vi "Dhoot_Sealed_side.vi"(0 "Calibrated Image":T3, 1 "Image In":T3(plugin-control), 2 "Centre X":dbl, 3 "Centre Y":dbl, 4 "Ref Edge ROI":T4, 5 "Ref Search Direction":u32(ring)=2 items=["Left to Right", "Right to Left", "Top to Bottom", "Bottom to Top"], 6 "Ref Edge Options":T7={"Edge Polarity"=2, "Kernel Size"=3, "Width"=3, "Minimum Edge Strength"=50.0, "Interpolation Type"=enum."Zero Order", "Data Processing Method"=enum."Average"} {"Edge Polarity" items=["All Edges", "Rising Edges", "Falling Edges"]; "Minimum Edge Strength" format="%.2f"; "Width" step=2; "Kernel Size" step=2}, 7 "error in (no error)":errorcluster, 8 "Meas ROI 1 [Before Transformation]":T2 {"Contours"."Type" items=["No Selection", "Point", "Line", "Rectangle", "Oval", "Polygon", "Freehand Region", "Annulus", "Unused2", "Unused3", "Broken Line", "Freehand Line", "Rotated Rectangle"]}, 9 "Ref Line Options":T5={"Number of Lines"=1, "Type"=enum."Best Edge Rake", "Min. Score"=10.0, "Max. Score"=1000.0, "Orientation"=0.0, "Angle Range"=50.0, "Angle Tolerance"=1.0, "Step Size"=3, "Min. SNR (db)"=0.0, "Min. Points (%)"=25.0, "Hough Iterations"=5} {"Min. Points (%)" min=0.0 max=100.0; "Min. SNR (db)" min=0.0; "Max. Score" min=0.0 max=1024.0; "Min. Score" min=0.0 max=1024.0 step=1.0}, 10 "ROI 1 Step Size":u32=5, 11 "Meas ROI 2 [Before Transformation]":T2 {"Contours"."Type" items=["No Selection", "Point", "Line", "Rectangle", "Oval", "Polygon", "Freehand Region", "Annulus", "Unused2", "Unused3", "Broken Line", "Freehand Line", "Rotated Rectangle"]}, 12 "ROI 1 Scan Direction":u16(ring) items=["Left To Right", "Right To Left", "Top To Bottom", "Bottom To Top"], 13 "ROI 2 Step Size":u32=5, 14 "ROI 1 Process":T9(ring)=enum."Get All Edges", 15 "ROI 2 Scan Direction":u16(ring) items=["Left To Right", "Right To Left", "Top To Bottom", "Bottom To Top"], 16 "ROI 1 Edge Options":T7={"Edge Polarity"=2, "Kernel Size"=3, "Width"=3, "Minimum Edge Strength"=50.0, "Interpolation Type"=enum."Zero Order", "Data Processing Method"=enum."Average"} {"Edge Polarity" items=["All Edges", "Rising Edges", "Falling Edges"]; "Minimum Edge Strength" format="%.2f"; "Width" step=2; "Kernel Size" step=2}, 17 "ROI 2 Process":T9(ring)=enum."Get All Edges", 18 "Overlay Enable":bool, 19 "ROI 2 Edge Options":T7={"Edge Polarity"=2, "Kernel Size"=3, "Width"=3, "Minimum Edge Strength"=50.0, "Interpolation Type"=enum."Zero Order", "Data Processing Method"=enum."Average"} {"Edge Polarity" items=["All Edges", "Rising Edges", "Falling Edges"]; "Minimum Edge Strength" format="%.2f"; "Width" step=2; "Kernel Size" step=2}) -> (21 "Side Length":sgl, 23 "Arrow Overlay lines":T1, 27 "error out":errorcluster)   [LabVIEW 2019, in "Algorithm.lvclass"]
uses:
  FrameworkOverrides/Algorithm.lvclass
  <vilib>/vision/NI_Vision_Development_Module.lvlib
  <vilib>/vision/Measure.llb/Edge Polarity.ctl
  <vilib>/vision/Measure.llb/Edge Options.ctl
  <vilib>/vision/Measure.llb/Straight Edge Process.ctl
  <vilib>/vision/Measure.llb/Straight Edge Options.ctl
  <vilib>/vision/Image Controls.llb/IMAQ Image.ctl
panel:
  out "max value 2":dbl
  out "max value":dbl
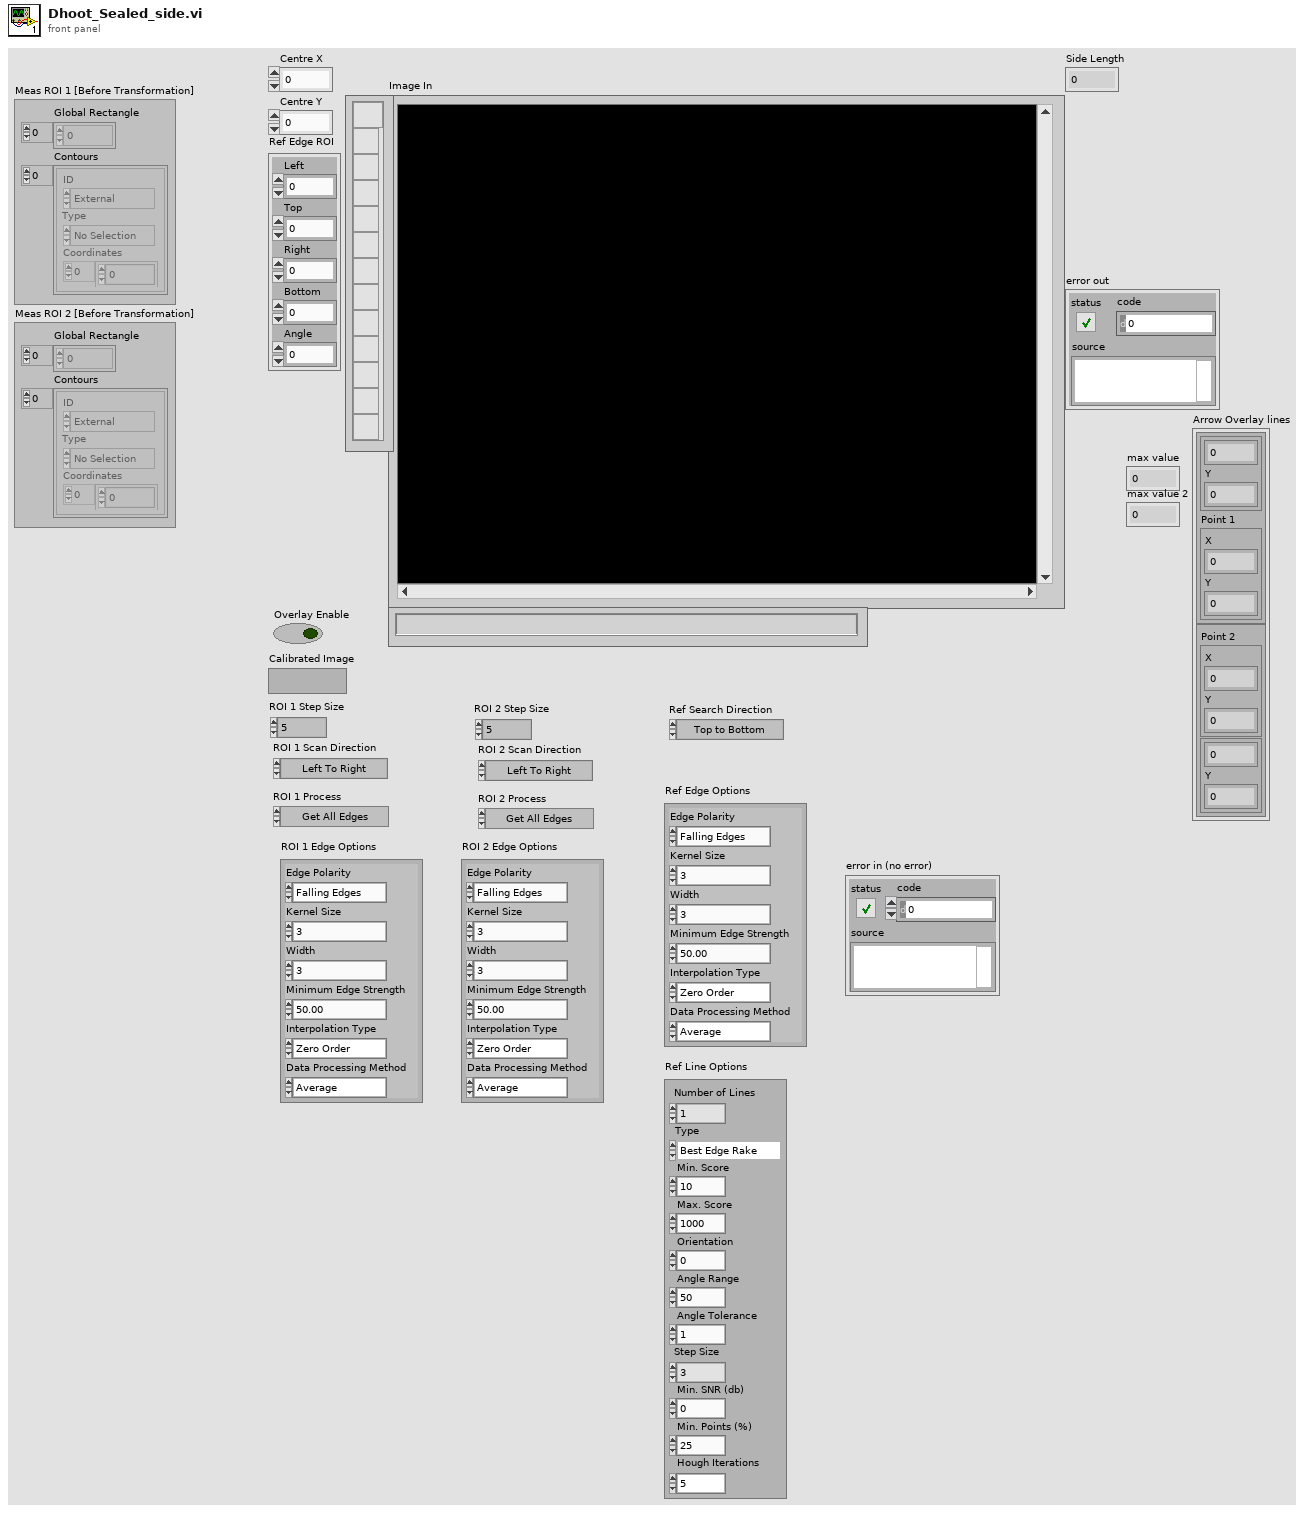
[diagram p1: front panel]
types:
  T1 = cluster{cluster{cluster{sgl, "Y":sgl}, "Point 1":cluster{"X":sgl, "Y":sgl}}, cluster{"Point 2":cluster{"X":sgl, "Y":sgl}, cluster{sgl, "Y":sgl}}}
  T2 = typedef "ROI Descriptor" = cluster{"Global Rectangle":i32[], "Contours":cluster{"ID":enum32{"External", "Internal"}, "Type":u32, "Coordinates":i32[]}[]}
  T3 = typedef "IMAQ Image.ctl" = refnum<image>
  T4 = cluster{"Left":dbl, "Top":dbl, "Right":dbl, "Bottom":dbl, "Angle":dbl}
  T5 = typedef "Straight Edge Options.ctl" = cluster{"Number of Lines":i32, "Type":T6, "Min. Score":dbl, "Max. Score":dbl, "Orientation":dbl, "Angle Range":dbl, "Angle Tolerance":dbl, "Step Size":u32, "Min. SNR (db)":dbl, "Min. Points (%)":dbl, "Hough Iterations":i32}
  T6 = typedef "Straight Edge Process.ctl" = enum32{"First Edge Rake", "Best Edge Rake", "Hough Edge Rake", "First Edge Projection", "Best Edge Projection"}
  T7 = typedef "Edge Options.ctl" = cluster{"Edge Polarity":T8, "Kernel Size":u32, "Width":u32, "Minimum Edge Strength":sgl, "Interpolation Type":enum32{"Zero Order", "Bilinear", "Quadratic", "Cubic", "Bilinear Fixed"}, "Data Processing Method":enum32{"Average", "Median"}}
  T8 = typedef "Edge Polarity.ctl" = u32
  T9 = enum16{"Get First Edge", "Get First + Last Edge", "Get All Edges", "Get Best Edge"}
  T10 = cluster{"Point1 (Pixels)":cluster{"X":sgl, "Y":sgl}, "Point2 (Pixels)":cluster{"X":sgl, "Y":sgl}, "Point1 (Real-World)":cluster{"X":sgl, "Y":sgl}, "Point2 (Real-World)":cluster{"X":sgl, "Y":sgl}, "Angle (Pixel)":dbl, "Angle (Real-World)":dbl, "Score":dbl, "Straightness":dbl, "Average SNR (db)":dbl, "Calibration Valid":bool}[]
  T11 = cluster{"Point1 (Pixels)":cluster{"X":sgl, "Y":sgl}, "Point2 (Pixels)":cluster{"X":sgl, "Y":sgl}, "Point1 (Real-World)":cluster{"X":sgl, "Y":sgl}, "Point2 (Real-World)":cluster{"X":sgl, "Y":sgl}, "Angle (Pixel)":dbl, "Angle (Real-World)":dbl, "Score":dbl, "Straightness":dbl, "Average SNR (db)":dbl, "Calibration Valid":bool}
  T12 = typedef "Edge New.ctl" = cluster{"Location (Pixel)":cluster{"X":sgl, "Y":sgl}, "Location (Real-World)":cluster{"X":sgl, "Y":sgl}, "Distance (Pixel)":dbl, "Distance (Real-World)":dbl, "Strength":dbl, "Noise":dbl, "Rising?":bool}
  T13 = typedef "Search Line.ctl" = cluster{"Start Point":cluster{"X":sgl, "Y":sgl}, "End Point":cluster{"X":sgl, "Y":sgl}, "Edge Info":T12[], "Edge Map":dbl[], "Calibration Valid":bool}
  T14 = cluster{"Point1 (Pixels)":cluster{"X":sgl, "Y":sgl}, "Point2 (Pixels)":cluster{"X":sgl, "Y":sgl}}
  T15 = cluster{"Point 1":cluster{"X":sgl, "Y":sgl}, "Point 2":cluster{"X":sgl, "Y":sgl}}
  T16 = cluster{cluster{sgl, "Y":sgl}, "Point 1":cluster{"X":sgl, "Y":sgl}}
  T17 = cluster{"Point 2":cluster{"X":sgl, "Y":sgl}, cluster{sgl, "Y":sgl}}
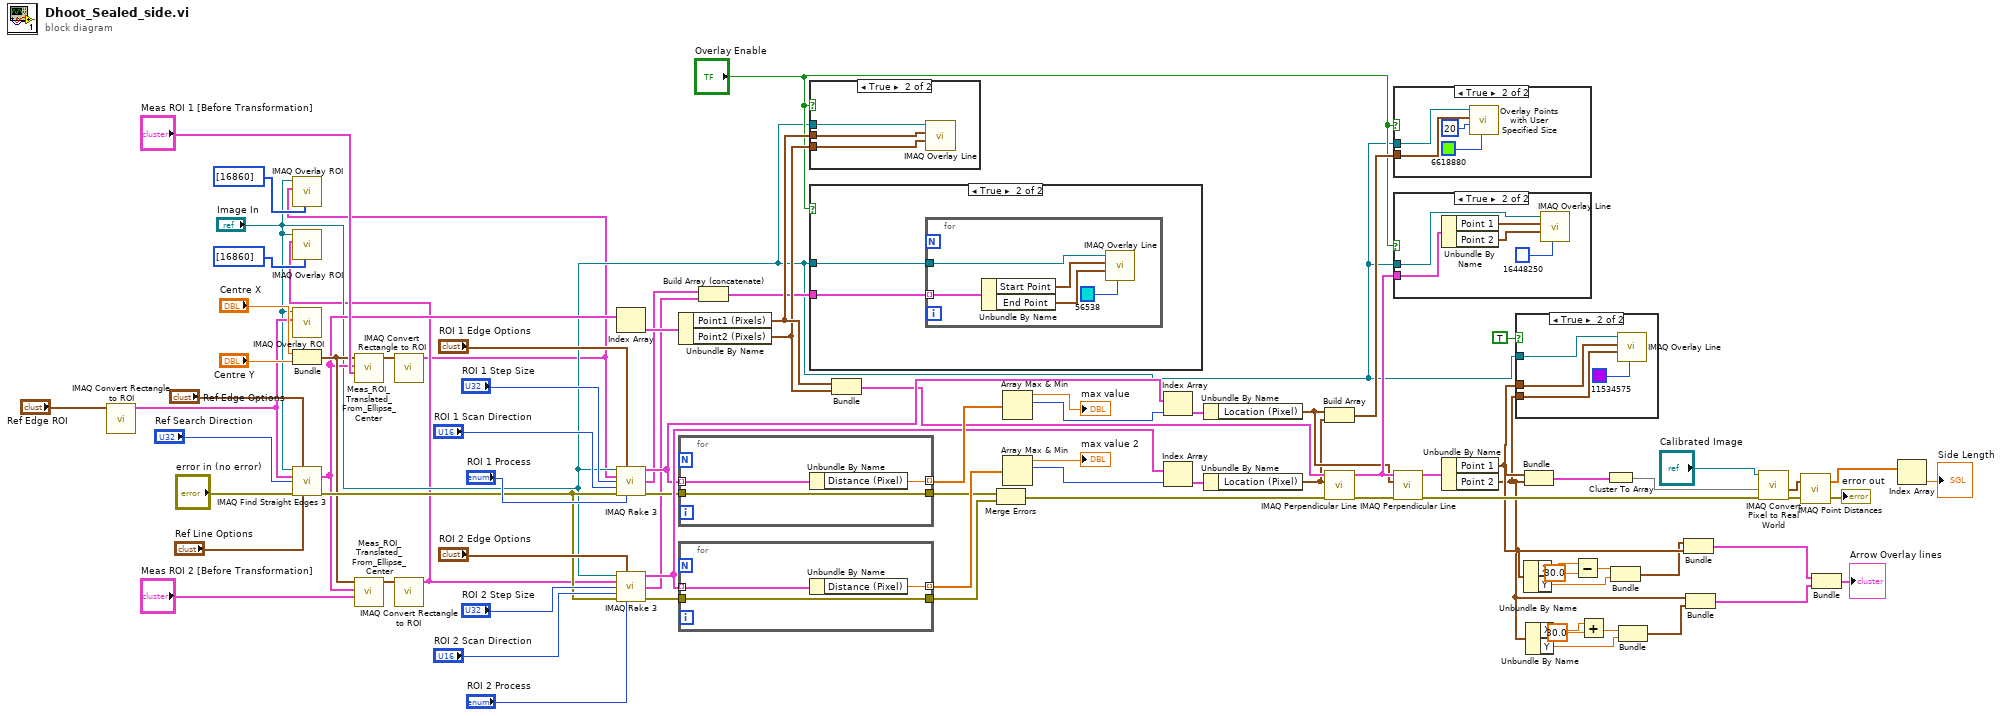
[diagram p0: block diagram]
diagram:
  n1 = call "IMAQ Convert Rectangle to ROI"("Rectangle"="Ref Edge ROI") -> ("ROI Descriptor"=w20:T2)  [unwired: 8 in, 1 out]
  n2 = call "IMAQ Overlay ROI"("ROI Descriptor"=w20, "Image"="Image In") -> ()  [unwired: 8 in, 2 out]
  n3 = Bundle("Centre X"="Centre X", "Centre Y"="Centre Y") -> (w26:cluster{"Centre X":dbl, "Centre Y":dbl})  [unwired: 1 in]
  n4 = call "IMAQ Find Straight Edges 3"("Image"="Image In", "Edge Options"="Ref Edge Options", "ROI Descriptor"=w20, "Search Direction"="Ref Search Direction", "error in (no error)"="error in (no error)", "Line Options"="Ref Line Options") -> ("Straight Edges"=w25:T10, "error out"=w30:errorcluster)  [unwired: 5 in, 3 out]
  n5 = call "Meas_ROI_Translated_From_Ellipse_Center.vi"("ROI Descriptor"="Meas ROI 1 [Before Transformation]", "Straight Edges"=w25, "Ellipse Center"=w26) -> ("Translated ROI"=w24:T4)  [unwired: 8 in]
  n6 = call "Meas_ROI_Translated_From_Ellipse_Center.vi"("ROI Descriptor"="Meas ROI 2 [Before Transformation]", "Straight Edges"=w25, "Ellipse Center"=w26) -> ("Translated ROI"=w23:T4)  [unwired: 8 in]
  n7 = call "IMAQ Convert Rectangle to ROI"("Rectangle"=w24) -> ("ROI Descriptor"=w17:T2)  [unwired: 8 in, 1 out]
  n8 = call "IMAQ Overlay ROI"("Colors (Green)"=u32[] [16860], "ROI Descriptor"=w17, "Image"="Image In") -> ()  [unwired: 7 in, 2 out]
  n9 = call "IMAQ Convert Rectangle to ROI"("Rectangle"=w23) -> ("ROI Descriptor"=w18:T2)  [unwired: 8 in, 1 out]
  n10 = call "IMAQ Overlay ROI"("Colors (Green)"=u32[] [16860], "ROI Descriptor"=w18, "Image"="Image In") -> ()  [unwired: 7 in, 2 out]
  n11 = Index Array(array=w25) -> (element=w57:T11)  [unwired: 1 in]
  n12 = call "IMAQ Rake 3"("Image"="Image In", "Edge Options"="ROI 1 Edge Options", "ROI Descriptor"=w17, "Step Size"="ROI 1 Step Size", "Scan Direction"="ROI 1 Scan Direction", "error in (no error)"=w30, "Process"="ROI 1 Process") -> ("First Edges"=w71:T12[], "Search Lines"=w48:T13[], "error out"=w66:errorcluster)  [unwired: 5 in, 1 out]
  n13 = call "IMAQ Rake 3"("Image"="Image In", "Edge Options"="ROI 2 Edge Options", "ROI Descriptor"=w18, "Step Size"="ROI 2 Step Size", "Scan Direction"="ROI 2 Scan Direction", "error in (no error)"=w30, "Process"="ROI 2 Process") -> ("First Edges"=w72:T12[], "Search Lines"=w47:T13[], "error out"=w65:errorcluster)  [unwired: 5 in, 1 out]
  n14 = Unbundle By Name(w57) -> ("Point1 (Pixels)"=w56:cluster{"X":sgl, "Y":sgl}, "Point2 (Pixels)"=w55:cluster{"X":sgl, "Y":sgl})
  n15 = for {
    tunnel: w71 -> [w85] mode=indexing
    tunnel: [w84] -> w74 mode=indexing
    tunnel: w66 -> [w83]
    tunnel: [w83] -> w64
    n16 = Unbundle By Name(w85) -> ("Distance (Pixel)"=w84:dbl)
  }
  n17 = for {
    tunnel: w72 -> [w88] mode=indexing
    tunnel: [w87] -> w73 mode=indexing
    tunnel: w65 -> [w86]
    tunnel: [w86] -> w63
    n18 = Unbundle By Name(w88) -> ("Distance (Pixel)"=w87:dbl)
  }
  n19 = Build Array (concatenate)(w48, w47) -> (w46:T13[])
  n20 = case shown="True" "Overlay Enable" {
    tunnel: w56 -> [_ w91]
    tunnel: w55 -> [_ w90]
    tunnel: "Image In" -> [_ w89]
    frame False {
    }
    frame True {
      n21 = call "IMAQ Overlay Line"("End Point"=w90, "Start Point"=w91, "Image"=w89) -> ()  [unwired: 7 in, 2 out]
    }
  }
  n22 = case shown="True" "Overlay Enable" {
    tunnel: w46 -> [_ w93]
    tunnel: "Image In" -> [_ w92]
    frame False {
    }
    frame True {
      n23 = for {
        tunnel: w93 -> [w98] mode=indexing
        tunnel: w92 -> [w94]
        n24 = Unbundle By Name(w98) -> ("Start Point"=w96:cluster{"X":sgl, "Y":sgl}, "End Point"=w95:cluster{"X":sgl, "Y":sgl})
        n25 = call "IMAQ Overlay Line"("Color"=u32 56538, "End Point"=w95, "Start Point"=w96, "Image"=w94) -> ()  [unwired: 6 in, 2 out]
      }
    }
  }
  n26 = Bundle("Point1 (Pixels)"=w56, "Point2 (Pixels)"=w55) -> (w51:T14)  [unwired: 1 in]
  n27 = Merge Errors(w64, w63) -> (w32:errorcluster)
  n28 = Array Max & Min(array=w74) -> (max value=→"max value":dbl, max index (indices)=w70:i32)  [unwired: 2 out]
  n29 = Array Max & Min(array=w73) -> (max value=→"max value 2":dbl, max index (indices)=w69:i32)  [unwired: 2 out]
  n30 = Index Array(array=w71, index=w70) -> (element=w68:T12)
  n31 = Index Array(array=w72, index=w69) -> (element=w67:T12)
  n32 = Unbundle By Name(w68) -> ("Location (Pixel)"=w50:cluster{"X":sgl, "Y":sgl})
  n33 = Unbundle By Name(w67) -> ("Location (Pixel)"=w49:cluster{"X":sgl, "Y":sgl})
  n34 = Build Array(w50, w49) -> (w60:cluster{"X":sgl, "Y":sgl}[])
  n35 = call "IMAQ Perpendicular Line"("error in (no error)"=w32, "Point"=w49, "Line"=w51) -> ("error out"=w52:errorcluster, "Perpendicular Line"=w54:T15)  [unwired: 6 in, 1 out]
  n36 = case shown="True" "Overlay Enable" {
    tunnel: w60 -> [_ w100]
    tunnel: "Image In" -> [_ w99]
    frame False {
    }
    frame True {
      n37 = call "Overlay Points with User Specified Size.vi"("Color"=u32 6618880, "Point Diameter (5)"=u32 20, "Points"=w100, "Image In"=w99) -> ()  [unwired: 6 in, 2 out]
    }
  }
  n38 = case shown="True" "Overlay Enable" {
    tunnel: w54 -> [_ w105]
    tunnel: "Image In" -> [_ w104]
    frame False {
    }
    frame True {
      n39 = Unbundle By Name(w105) -> ("Point 1"=w107:cluster{"X":sgl, "Y":sgl}, "Point 2"=w106:cluster{"X":sgl, "Y":sgl})
      n40 = call "IMAQ Overlay Line"("Color"=u32 16448250, "End Point"=w106, "Start Point"=w107, "Image"=w104) -> ()  [unwired: 6 in, 2 out]
    }
  }
  n41 = call "IMAQ Perpendicular Line"("error in (no error)"=w52, "Point"=w50, "Line"=w54) -> ("error out"=w37:errorcluster, "Perpendicular Line"=w53:T15)  [unwired: 6 in, 1 out]
  n42 = Unbundle By Name(w53) -> ("Point 1"=w15:cluster{"X":sgl, "Y":sgl}, "Point 2"=w9:cluster{"X":sgl, "Y":sgl})
  n43 = case shown="True" TRUE {
    tunnel: "Image In" -> [_ w111]
    tunnel: w15 -> [_ w110]
    tunnel: w9 -> [_ w109]
    frame False {
    }
    frame True {
      n44 = call "IMAQ Overlay Line"("Color"=u32 11534575, "End Point"=w109, "Start Point"=w110, "Image"=w111) -> ()  [unwired: 6 in, 2 out]
    }
  }
  n45 = Unbundle By Name(w15) -> ("X"=w14:sgl, "Y"=w11:sgl)
  n46 = Bundle("Point 1"=w15, "Point 2"=w9) -> (w43:T15)  [unwired: 1 in]
  n47 = Unbundle By Name(w9) -> ("X"=w8:sgl, "Y"=w5:sgl)
  n48 = Subtract(x=w14, y=sgl 30.0) -> (x-y=w12:sgl)
  n49 = Add(x=w8, y=sgl 30.0) -> (x+y=w6:sgl)
  n50 = Cluster To Array(cluster=w43) -> (array=w42:cluster{"X":sgl, "Y":sgl}[])
  n51 = Bundle(w12, "Y"=w11) -> (w10:cluster{sgl, "Y":sgl})  [unwired: 1 in]
  n52 = Bundle(w6, "Y"=w5) -> (w4:cluster{sgl, "Y":sgl})  [unwired: 1 in]
  n53 = Bundle(w10, "Point 1"=w15) -> (w3:T16)  [unwired: 1 in]
  n54 = Bundle("Point 2"=w9, w4) -> (w2:T17)  [unwired: 1 in]
  n55 = call "IMAQ Convert Pixel to Real World"("error in (no error)"=w37, "Array of Pixel Coordinates"=w42, "Calibrated Image"="Calibrated Image") -> ("error out"=w36:errorcluster, "Array of Real World Coordinates"=w41:cluster{"X":sgl, "Y":sgl}[])  [unwired: 3 in, 4 out]
  n56 = call "IMAQ Point Distances"("Points"=w41, "error in (no error)"=w36) -> ("Distances"=w39:sgl[], "error out"=→"error out":errorcluster)  [unwired: 3 in]
  n57 = Bundle(w3, w2) -> (→"Arrow Overlay lines":T1)  [unwired: 1 in]
  n58 = Index Array(array=w39) -> (element=→"Side Length":sgl)  [unwired: 1 in]
